vi "Test PowerShell.vi"   [LabVIEW 2016]
uses:
  <vilib>/addons/_JKI Toolkits/Caraya/classes/Test/Test.lvclass
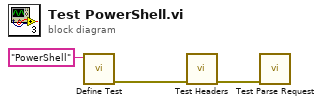
[diagram p0: block diagram]
diagram:
  n1 = call <vilib>:"Define Test.vi"("Label (VI Title)"="PowerShell") -> ("error out"=w2:errorcluster)  [unwired: 10 in]
  n2 = call "Test Headers.vi"("error in"=w2) -> ("error out"=w1:errorcluster)  [unwired: 10 in]
  n3 = call "Test Parse Request.vi"("error in (no error)"=w1) -> ()  [unwired: 10 in, 1 out]
